vi "Init.vi"(8 "error in (no error)":errorcluster, 11 "Data in":refnum<class "UI-Bus.lvclass">) -> (0 "error out":errorcluster, 3 "Data out":refnum<class "UI-Bus.lvclass">)   [LabVIEW 2021, in "UI-Bus.lvclass"]
doc: "Abstract Data Classes 2.1.1.12\nTim Streeter - TSA\nCopyright (c) 2024, TSAOmni-Bus 2.0.1.6\nTim - TSA\nCopyright (c) 2024, TSA"
uses:
  UI-Bus.lvclass
  C:/Program Files (x86)/National Instruments/LabVIEW 2021/vi.lib/TSA/Omni-Bus/Omni-Bus/Bus Access/Bus_Access.lvclass
  <vilib>/TSA/Omni-Bus/Omni-Bus/Bus Access/Bus_Access.lvclass/Bus_Access.ctl
  UI-Bus.lvclass/UI-Bus.ctl
  <vilib>/TSA/Omni-Bus/Omni-Bus/Bus Access/Properties/Read Tag Root.vi
  <vilib>/TSA/Omni-Bus/Omni-Bus/Bus Access/Properties/Write Values.vi
  <vilib>/TSA/Omni-Bus/Omni-Bus/Bus Access/Properties/Write Tags.vi
  <vilib>/TSA/Abstract Data Classes/Abs_Types/Type/Abs_Type.lvclass
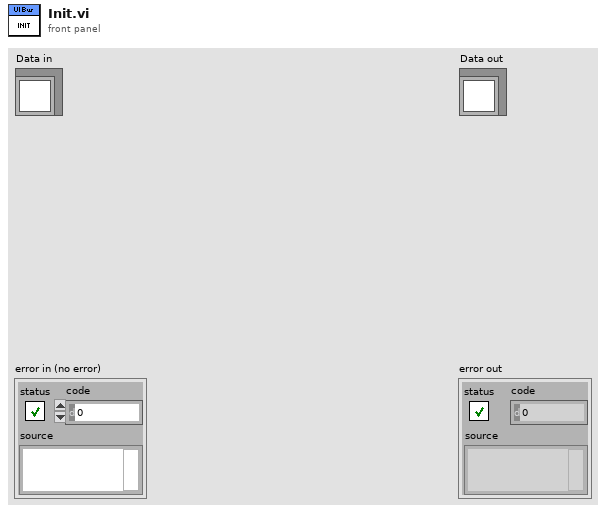
[diagram p1: front panel]
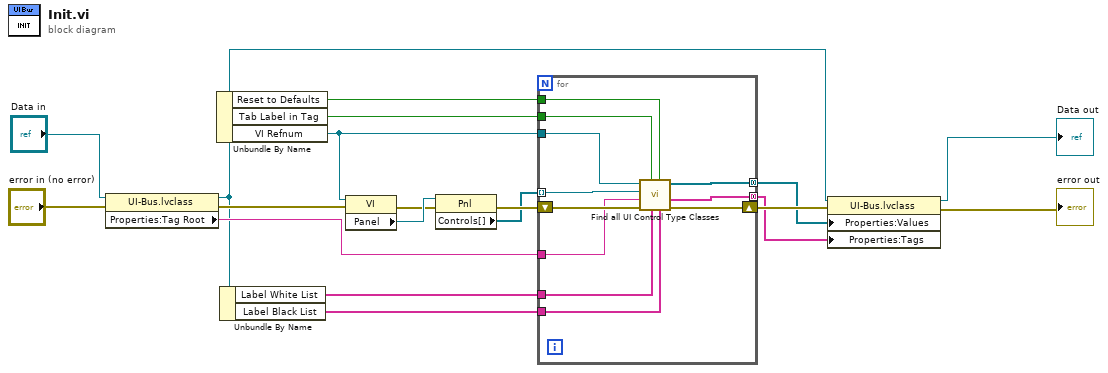
[diagram p0: block diagram]
diagram:
  n1 = property class="UI-Bus.lvclass"(reference="Data in", error in="error in (no error)") -> (reference out=w5:refnum<class "UI-Bus.lvclass">, error out=w12:errorcluster, "Properties:Tag Root"=w11:string)
  n2 = Unbundle By Name(w5) -> ("Reset to Defaults"=w1:bool, "Tab Label in Tag"=w2:bool, "VI Refnum"=w15:refnum<vi>)
  n3 = Unbundle By Name(w5) -> ("Label White List"=w4:string[], "Label Black List"=w3:string[])
  n4 = property class="VI"(reference=w15, error in=w12) -> (error out=w18:errorcluster, "Panel"=w19:refnum<vi>)  [unwired: 1 out]
  n5 = property class="Pnl"(reference=w19, error in=w18) -> (error out=w17:errorcluster, "Controls[]"=w16:refnum<vi>[])  [unwired: 1 out]
  n6 = for {
    shift-right: [w26] -> w10
    shift-left: w17 -> [w30]
    tunnel: w16 -> [w29] mode=indexing
    tunnel: w15 -> [w28]
    tunnel: [w27] -> w9 mode=concatenating
    tunnel: w11 -> [w25]
    tunnel: [w24] -> w8 mode=concatenating
    tunnel: w4 -> [w23]
    tunnel: w3 -> [w22]
    tunnel: w2 -> [w21]
    tunnel: w1 -> [w20]
    n7 = call "Find all UI Control Type Classes.vi"("Label Black List"=w22, "Reset to Defaults"=w20, "Label White List"=w23, "Tab Label in Tag?"=w21, "error in (no error)"=w30, "Root Label"=w25, "Ctl Refnum"=w29, "VI in"=w28) -> ("error out"=w26:errorcluster, "Labels"=w24:string[], "Values"=w27:refnum<class "Abs_Type.lvclass">[])  [unwired: 1 in]
  }
  n8 = property class="UI-Bus.lvclass"(reference=w5, error in=w10, "Properties:Values"=w9, "Properties:Tags"=w8) -> (reference out=→"Data out":refnum<class "UI-Bus.lvclass">, error out=→"error out":errorcluster)
